vi "DriveModuleControl_TravTuneKa.vi"(8 "error in":errorcluster, 9 "Actual State":T1={"Speed"=0.0, "Angle"={"VALUE"=0.0, "COS"=1.0, "SIN"=0.0}} {"Angle"."SIN" format="%13.4f"; "Angle"."COS" format="%13.4f"; "Angle"."VALUE" format="%13.4f"}, 10 "Desired State":T1={"Speed"=0.0, "Angle"={"VALUE"=0.0, "COS"=1.0, "SIN"=0.0}} {"Angle"."SIN" format="%13.4f"; "Angle"."COS" format="%13.4f"; "Angle"."VALUE" format="%13.4f"}, 11 "ModualNamePrefix":i32) -> (0 "error out":errorcluster)   [LabVIEW 2023]
uses:
  <vilib>/Rock Robotics/WPI/ThirdParty/JAS_Junk/TrajLib/TypeDef/SWERVE_DRIVE_MODULE_STATE.ctl
  <vilib>/Rock Robotics/WPI/ThirdParty/JAS_Junk/TrajLib/TypeDef/ROTATION2D.ctl
  <vilib>/Rock Robotics/WPI/ThirdParty/JAS_Junk/TrajLib/Rotation2d_Minus.vi
  <vilib>/Rock Robotics/WPI/ThirdParty/JAS_Junk/TrajLib/Rotation2d_GetRadians.vi
  <vilib>/Rock Robotics/WPI/ThirdParty/JAS_Junk/TrajLib/SwerveModuleState_New.vi
  <vilib>/Rock Robotics/WPI/ThirdParty/JAS_Junk/TrajLib/Rotation2d_RotateBy.vi
  <vilib>/Rock Robotics/WPI/ThirdParty/JAS_Junk/TrajLib/Rotation2d_CreateAngle.vi
  <vilib>/Rock Robotics/WPI/ThirdParty/JAS_Junk/TrajLib/SimpleMotorFF_Calculate.vi
  <vilib>/Rock Robotics/WPI/ThirdParty/JAS_Junk/TrajLib/PIDController_AtSetpoint.vi
  <vilib>/Rock Robotics/WPI/ThirdParty/JAS_Junk/TrajLib/PIDController_SetPIDF.vi
  <vilib>/Rock Robotics/WPI/ThirdParty/JAS_Junk/TrajLib/PIDController_SetDerivativeFilter.vi
  <vilib>/Rock Robotics/WPI/ThirdParty/JAS_Junk/TrajLib/PIDController_SetIntegratorRange.vi
  <vilib>/Rock Robotics/WPI/ThirdParty/JAS_Junk/TrajLib/PIDController_SetTolerancePandV.vi
  <vilib>/Rock Robotics/WPI/ThirdParty/JAS_Junk/TrajLib/PIDController_DisableContinousInput.vi
  <vilib>/Rock Robotics/WPI/ThirdParty/JAS_Junk/TrajLib/PIDController_EnableContinousInput.vi
  <vilib>/Rock Robotics/WPI/ThirdParty/JAS_Junk/TrajLib/PIDController_Reset.vi
  <vilib>/Rock Robotics/WPI/ThirdParty/JAS_Junk/TrajLib/PIDController_New.vi
  <vilib>/Rock Robotics/WPI/ThirdParty/JAS_Junk/TrajLib/PIDController_SetOutputLimits.vi
  <vilib>/Rock Robotics/WPI/ThirdParty/JAS_Junk/TrajLib/VI/PIDController_SetIntegratorZone.vi
  <vilib>/Rock Robotics/WPI/ThirdParty/JAS_Junk/TrajLib/Rotation2d_UnaryMinus.vi
  <vilib>/Rock Robotics/WPI/ThirdParty/JAS_Junk/TrajLib/Rotation2d_CreateXY.vi
  <vilib>/Rock Robotics/WPI/ThirdParty/JAS_Junk/TrajLib/PIDController_NewPeriod.vi
  <vilib>/Rock Robotics/WPI/ThirdParty/JAS_Junk/TrajLib/Util_CalcDist.vi
  <vilib>/Rock Robotics/SystemInterfaces/NetworkCommunication/NetComm_UsageReport_report.vi
  DriveGlobal.vi
  <vilib>/Rock Robotics/WPI/ThirdParty/Phoenix6/Phoenix6_Device_RefNumRegistryGet.vi
  <vilib>/Rock Robotics/WPI/MotorControl/WPI_MotorControlRefNum Registry Get.vi
  <vilib>/Rock Robotics/Network Tables/NT Write Number.vi
  <vilib>/Rock Robotics/WPI/ThirdParty/JAS_Junk/TrajLib/Globals/Util_LibraryGlobals.vi
  <vilib>/Rock Robotics/WPI/ThirdParty/JAS_Junk/TrajLib/PIDController_AdvCalculate_FF_Sp_Pv.vi
  DriveTuningGlobals.vi
  <vilib>/Rock Robotics/Network Tables/NT Write Boolean.vi
  <vilib>/Rock Robotics/WPI/ThirdParty/JAS_Junk/TrajLib/Trajectory_Library.lvlib
  <vilib>/Rock Robotics/WPI/ThirdParty/REV Robotics/REVLib/Typedef/Spark MAX Control Type.ctl
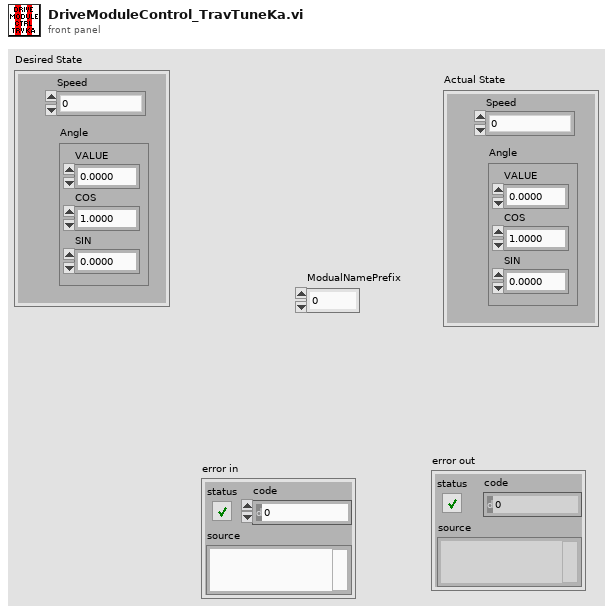
[diagram p1: front panel]
types:
  T1 = typedef "Trajectory_Library.lvlib/SWERVE_DRIVE_MODULE_STATE.ctl" = cluster{"Speed":dbl, "Angle":T2}
  T2 = typedef "Trajectory_Library.lvlib/ROTATION2D.ctl" = cluster{"VALUE":dbl, "COS":dbl, "SIN":dbl}
  T3 = typedef "Spark MAX Control Type.ctl" = enum16{"Percent VBus", "Voltage", "Velocity", "Position", "Smart Motion", "Current", "Smart Velocity", "MAXMotion Position", "MAXMotion Velocity"}
  T4 = typedef "WPI_MotorControlDeviceRef.ctl" = cluster{"DeviceStatus":errorcluster, "Type":T5, "PWM":cluster{"PWM Channel":T6, "DeadBand":T7}, "CAN":cluster{"Device Number":u8, "SetOutput VI Ref":variant, "GetOutput VI Ref":variant, "Enable VI Ref":variant, "Disable VI Ref":variant, "Data":variant}, "Invert":bool, "DIO PWM":cluster{"PWM \"Enable\" Channel":T6, "DIOChannel":T8, "PWM Rate":dbl}}
  T5 = typedef "WPI_MotorControlType.ctl" = enum16{"PWM", "CAN", "DIO PWM"}
  T6 = typedef "FPGA_DIOPWMChannel.ctl" = enum8{"PWM 0", "PWM 1", "PWM 2", "PWM 3", "PWM 4", "PWM 5", "PWM 6", "PWM 7", "PWM 8", "PWM 9", "PWM MXP 0", "PWM MXP 1", "PWM MXP 2", "PWM MXP 3", "PWM MXP 4", "PWM MXP 5", "PWM MXP 6", "PWM MXP 7", "PWM MXP 8", "PWM MXP 9", "Invalid"}
  T7 = typedef "WPI_PWMDeadband.ctl" = cluster{"Name":string, "maxPositivePwm":i32, "minPositivePwm":i32, "centerPwm":i32, "maxNegativePwm":i32, "minNegativePwm":i32, "angularRange":u16}
  T8 = typedef "FPGA_DIOChannel.ctl" = enum8{"DIO 0", "DIO 1", "DIO 2", "DIO 3", "DIO 4", "DIO 5", "DIO 6", "DIO 7", "DIO 8", "DIO 9", "DIO MXP 0", "DIO MXP 1", "DIO MXP 2", "DIO MXP 3", "DIO MXP 4", "DIO MXP 5", "DIO MXP 6", "DIO MXP 7", "DIO MXP 8", "DIO MXP 9", "DIO MXP 10", "DIO MXP 11", "DIO MXP 12", "DIO MXP 13", "DIO MXP 14", "DIO MXP 15", "SPI Port CS1", "SPI Port CS2", "SPI Port CS3", "SPI Port MISO", "SPI Port MOSI", "Invalid"}
  T9 = typedef "Trajectory_Library.lvlib/SIMPLE_MOTOR_FF.ctl" = cluster{"Ks":dbl, "Kv":dbl, "Ka":dbl, "KnInv":dbl}
  T10 = typedef "Trajectory_Library.lvlib/PID_ADV_LIMITS.ctl" = cluster{"MaxInput":dbl, "MinInput":dbl, "Continuous":bool, "MaxOutput":dbl, "MinOutput":dbl}
  T11 = typedef "Trajectory_Library.lvlib/PID_ADV_TUNING.ctl" = cluster{"Kf":dbl, "Kp":dbl, "Ki":dbl, "Kd":dbl, "MaximumIntegral":dbl, "MinimumIntegral":dbl, "Filter Derivative":bool, "IntegralZone":dbl}
  T12 = typedef "Trajectory_Library.lvlib/SIMPLE_MOTOR_FF_KA_TUNE_PARAMS.ctl" = cluster{"Max SP":dbl, "Min Eval SP":dbl, "Max Eval SP":dbl, "Ramp Rate":dbl}
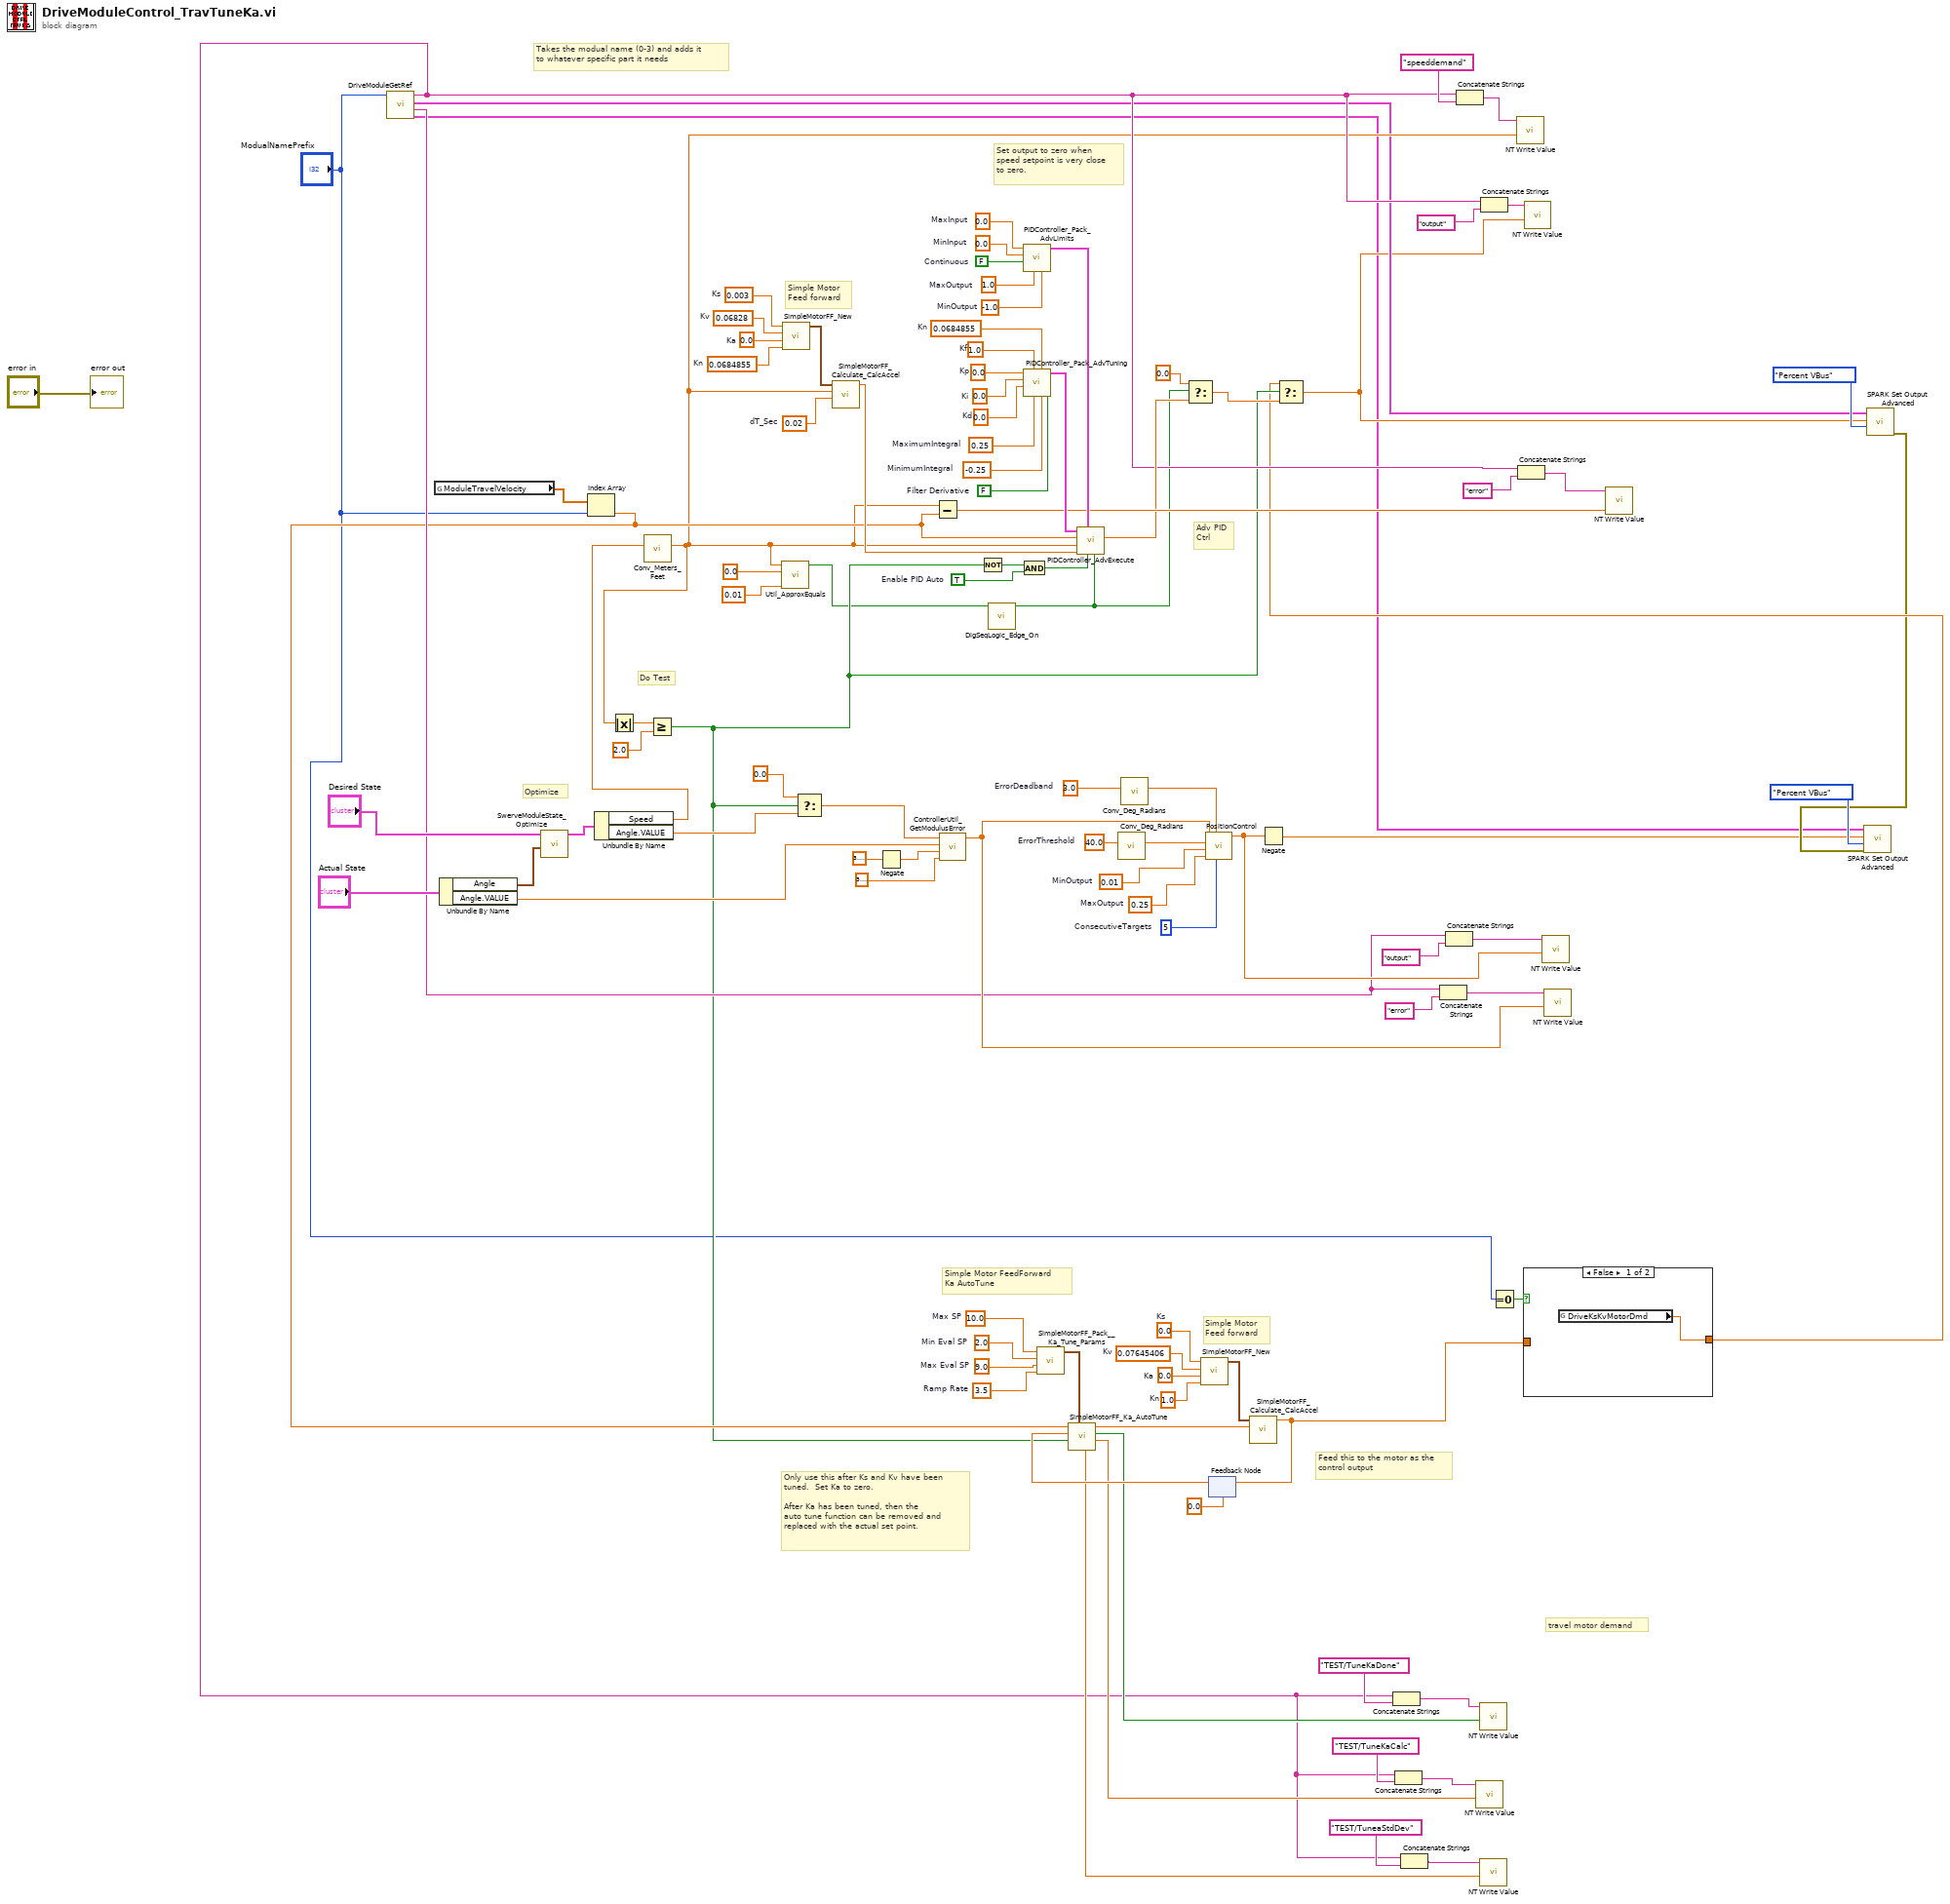
[diagram p0: block diagram]
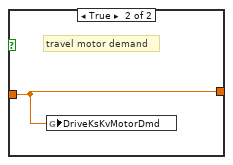
[diagram p2: hidden frame]
diagram:
  w36 = 1.0  # Kn
  w34 = 0.0  # Ks
  w33 = 0.07645406  # Kv
  w32 = 0.0  # Ka
  w31 = 10.0  # Max SP
  w30 = 2.0  # Min Eval SP
  w29 = 9.0  # Max Eval SP
  w28 = 3.5  # Ramp Rate
  w49 = TRUE  # Enable PID Auto
  w58 = 0.0684855  # Kn
  w74 = 0.0  # Kp
  w73 = 0.0  # Ki
  w72 = 0.0  # Kd
  w71 = 1.0  # Kf
  w70 = 0.25  # MaximumIntegral
  w69 = -0.25  # MinimumIntegral
  w68 = FALSE  # Filter Derivative
  w66 = 0.0  # MinInput
  w65 = FALSE  # Continuous
  w64 = 1.0  # MaxOutput
  w67 = -1.0  # MinOutput
  w63 = 0.0  # MaxInput
  w80 = 0.0684855  # Kn
  w79 = 0.02  # dT_Sec
  w77 = 0.003  # Ks
  w76 = 0.06828  # Kv
  w75 = 0.0  # Ka
  w89 = 5  # ConsecutiveTargets
  w86 = 0.25  # MaxOutput
  w90 = 0.01  # MinOutput
  w83 = 40.0  # ErrorThreshold
  w85 = 3.0  # ErrorDeadband
  # "Only use this after Ks and Kv have been\ntuned.  Set Ka to zero.\n\nAfter Ka has been tuned, then the \nauto tune function can be removed and\nreplaced with the actual set point."
  # "Feed this to the motor as the\ncontrol output"
  # "Simple Motor\nFeed forward"
  # "Simple Motor FeedForward\nKa AutoTune"
  # "travel motor demand"
  # "Do Test"
  # "Optimize"
  # "Set output to zero when\nspeed setpoint is very close\nto zero."
  # "Adv PID\nCtrl"
  # "Simple Motor\nFeed forward"
  # "Takes the modual name (0-3) and adds it \nto whatever specific part it needs"
  n1 = call "DriveModuleGetRef.vi"("ModualNamePrefix"="ModualNamePrefix") -> ("SpinMot"=w2:T4, "SpinStr"=w54:string, "TravMot"=w4:T4, "TravStr"=w16:string)  [unwired: 5 in, 2 out]
  n2 = global read "DriveGlobal.vi" "ModuleTravelVelocity"() -> (w59:dbl[])
  n3 = Unbundle By Name("Actual State") -> ("Angle"=w96:T2, "Angle.VALUE"=w93:dbl)
  n4 = call <vilib>:"SwerveModuleState_Optimize.vi"("CurrentAngle"=w96, "Desired State"="Desired State") -> ("out SWERVE_DRIVE_MODULE_STATE"=w94:T1)  [unwired: 9 in]
  n5 = Index Array(array=w59, index="ModualNamePrefix") -> (element=w23:dbl)
  n6 = Unbundle By Name(w94) -> ("Speed"=w46:dbl, "Angle.VALUE"=w43:dbl)
  n7 = call <vilib>:"Conv_Meters_Feet.vi"("Meters"=w46) -> ("Feet"=w14:dbl)  [unwired: 10 in]
  n8 = Absolute Value(x=w14) -> (abs(x)=w45:dbl)
  n9 = Greater Or Equal?(x=w45, y=2.0) -> (x >= y?=w15:bool)
  n10 = call <vilib>:"Util_ApproxEquals.vi"("Tolerance"=0.01, "Value 2"=0.0, "Value 1"=w14) -> ("ApproxEquals"=w9:bool)  [unwired: 8 in]
  n11 = call <vilib>:"SimpleMotorFF_New.vi"("Kn"=w80, "Ka"=w75, "Kv"=w76, "Ks"=w77) -> ("SIMPLE_MOTOR_FF"=w78:T9)  [unwired: 7 in]
  n12 = Select(t=0.0, s=w15, f=w43) -> (s? t:f=w40:dbl)
  n13 = call <vilib>:"SimpleMotorFF_Calculate_CalcAccel.vi"("dT_Sec"=w79, "VelSp"=w14, "SIMPLE_MOTOR_FF"=w78) -> ("FeedForward"=w60:dbl)  [unwired: 8 in]
  n14 = Negate(x=3.141592653589793) -> (-x=w95:dbl)
  n15 = Subtract(x=w14, y=w23) -> (x-y=w55:dbl)
  n16 = call <vilib>:"ControllerUtil_GetModulusError.vi"("Maximum_Input"=3.141592653589793, "Minimum_Input"=w95, "Measurerment(PV)"=w93, "Reference(SP)"=w40) -> ("Error"=w87:dbl)  [unwired: 7 in]
  n17 = Not(x=w15) -> (.not. x?=w50:bool)
  n18 = call <vilib>:"DigSeqLogic_Edge_On.vi"("Input"=w9) -> ("On Edge"=w8:bool)  [unwired: 10 in]
  n19 = And(x=w50, y=w49) -> (x .and. y?=w51:bool)
  n20 = call <vilib>:"PIDController_Pack_AdvLimits.vi"("MinOutput"=w67, "MaxOutput"=w64, "Continuous"=w65, "MinInput"=w66, "MaxInput"=w63) -> ("Adv PID Limits"=w61:T10)  [unwired: 6 in]
  n21 = call <vilib>:"PIDController_Pack_AdvTuning.vi"("Filter Derivative"=w68, "MinimumIntegral"=w69, "Kn"=w58, "MaximumIntegral"=w70, "Kf"=w71, "Kd"=w72, "Ki"=w73, "Kp"=w74) -> ("Adv PID Tuning"=w62:T11)  [unwired: 3 in]
  n22 = call <vilib>:"SimpleMotorFF_Pack__Ka_Tune_Params.vi"("Ramp Rate"=w28, "Max Eval SP"=w29, "Min Eval SP"=w30, "Max SP"=w31) -> ("Packed Params"=w27:T12)  [unwired: 7 in]
  n23 = call <vilib>:"PIDController_AdvExecute.vi"("Reset"=w8, "Auto"=w51, "Adv PID Limits"=w61, "FF-FeedForward"=w60, "SP-SetPoint"=w14, "PV-Measurement"=w23, "Adv PID Tuning"=w62) -> ("CO-ControlOutput"=w48:dbl)  [unwired: 2 in, 2 out]
  n24 = call <vilib>:"Conv_Deg_Radians.vi"("Degress"=w83) -> ("Radians"=w82:dbl)  [unwired: 10 in]
  n25 = call <vilib>:"Conv_Deg_Radians.vi"("Degress"=w85) -> ("Radians"=w84:dbl)  [unwired: 10 in]
  n26 = Select(t=0.0, s=w8, f=w48) -> (s? t:f=w41:dbl)
  n27 = call <vilib>:"SimpleMotorFF_New.vi"("Kn"=w36, "Ka"=w32, "Kv"=w33, "Ks"=w34) -> ("SIMPLE_MOTOR_FF"=w35:T9)  [unwired: 7 in]
  n28 = call "PositionControl.vi"("ConsecutiveTargets"=w89, "ErrorDeadband"=w84, "MaxOutput"=w86, "MinOutput"=w90, "ErrorThreshold"=w82, "Error"=w87) -> ("OutputValue"=w81:dbl)  [unwired: 3 in, 2 out]
  n29 = feedback #1(0.0 ("FeedForward")) -> (w38:dbl)
  n30 = call <vilib>:"SimpleMotorFF_Ka_AutoTune.vi"("SimpleMotorFeedforward_KaTune_Pack"=w27, "Run Test"=w15, "CO Control Output"=w38, "PV ProcessVariable"=w23) -> ("Ka Calc"=w25:dbl, "Test Complete"=w26:bool, "SP Setpoint"=w37:dbl, "Ka StdDev"=w24:dbl)  [unwired: 1 in, 3 out]
  n31 = call <vilib>:"SimpleMotorFF_Calculate_CalcAccel.vi"("VelSp"=w37, "SIMPLE_MOTOR_FF"=w35) -> ("FeedForward"=w12:dbl)  [unwired: 9 in]
  n32 = feedback-in #1(w12) -> ()
  n33 = Negate(x=w81) -> (-x=w1:dbl)
  n34 = Concatenate Strings(w16, "TEST/TuneKaDone" ("name")) -> (w19:string)
  n35 = Concatenate Strings(w16, "TEST/TuneKaCalc" ("name")) -> (w18:string)
  n36 = Concatenate Strings(w16, "TEST/TuneaStdDev" ("name")) -> (w17:string)
  n37 = Concatenate Strings(w54, "error" ("refnum name")) -> (w100:string)
  n38 = Concatenate Strings(w54, "output" ("refnum name")) -> (w88:string)
  n39 = Concatenate Strings(w16, "speeddemand" ("refnum name")) -> (w104:string)
  n40 = call-poly <vilib>:"NT Write Value.vi"("value"=w25, "name"=w18) -> ()  [unwired: 9 in, 1 out]
  n41 = call-poly <vilib>:"NT Write Value.vi"("value"=w26, "name"=w19) -> ()  [unwired: 9 in, 1 out]
  n42 = call-poly <vilib>:"NT Write Value.vi"("value"=w24, "name"=w17) -> ()  [unwired: 9 in, 1 out]
  n43 = Concatenate Strings(w16, "output" ("refnum name")) -> (w102:string)
  n44 = Equal To 0?(x="ModualNamePrefix") -> (x = 0?=w13:bool)
  n45 = call-poly <vilib>:"NT Write Value.vi"("value"=w14, "name"=w104) -> ()  [unwired: 9 in, 1 out]
  n46 = Concatenate Strings(w16, "error" ("refnum name")) -> (w56:string)
  n47 = case shown="False" w13 {
    tunnel: w12 -> [_ w108]
    tunnel: [w107 w108] -> w11
    frame False {
      n48 = global read "DriveTuningGlobals.vi" "DriveKsKvMotorDmd"() -> (w107:dbl)
    }
    frame True {
      # "travel motor demand"
      n49 = global write "DriveTuningGlobals.vi" "DriveKsKvMotorDmd"(w108) -> ()
    }
  }
  n50 = Select(t=w11, s=w15, f=w41) -> (s? t:f=w3:dbl)
  n51 = call-poly <vilib>:"NT Write Value.vi"("value"=w3, "name"=w102) -> ()  [unwired: 9 in, 1 out]
  n52 = call-poly <vilib>:"NT Write Value.vi"("value"=w81, "name"=w88) -> ()  [unwired: 9 in, 1 out]
  n53 = call-poly <vilib>:"NT Write Value.vi"("value"=w87, "name"=w100) -> ()  [unwired: 9 in, 1 out]
  n54 = call-poly <vilib>:"NT Write Value.vi"("value"=w55, "name"=w56) -> ()  [unwired: 9 in, 1 out]
  n55 = call <vilib>:"SPARK Set Output Advanced.vi"("Control Mode"=Spark_MAX_Control_Type."Percent VBus", "Setpoint"=w3, "MotorControlDevRef"=w4) -> ("error out"=w5:errorcluster)  [unwired: 7 in, 1 out]
  n56 = call <vilib>:"SPARK Set Output Advanced.vi"("error in (no error)"=w5, "Control Mode"=Spark_MAX_Control_Type."Percent VBus", "Setpoint"=w1, "MotorControlDevRef"=w2) -> ()  [unwired: 6 in, 2 out]
  "error out" <- "error in"
